vi "split and resample.vi"(9 "real zero index":i32=225, 10 "B field array":dbl[](array[numeric]), 11 "cond":T1(graph)) -> (0 "resampled number of curves":i32, 1 "new B field\noffset and multiplier":cluster{"N1":dbl, dbl}, 2 "resampled B":dbl[](array[numeric]), 3 "resampled cond":T1(graph))   [LabVIEW 2016, in "Tranconductance SM.lvclass"]
uses:
  Tranconductance SM.lvclass
  <userlib>/LevyLab/XY Utilities/Typedefs/Interpolation Configuration--cluster.ctl
  <userlib>/LevyLab/XY Utilities/subVIs/Interpolate (single).vi
  <userlib>/LevyLab/XY Utilities/xy_utilities.lvlib
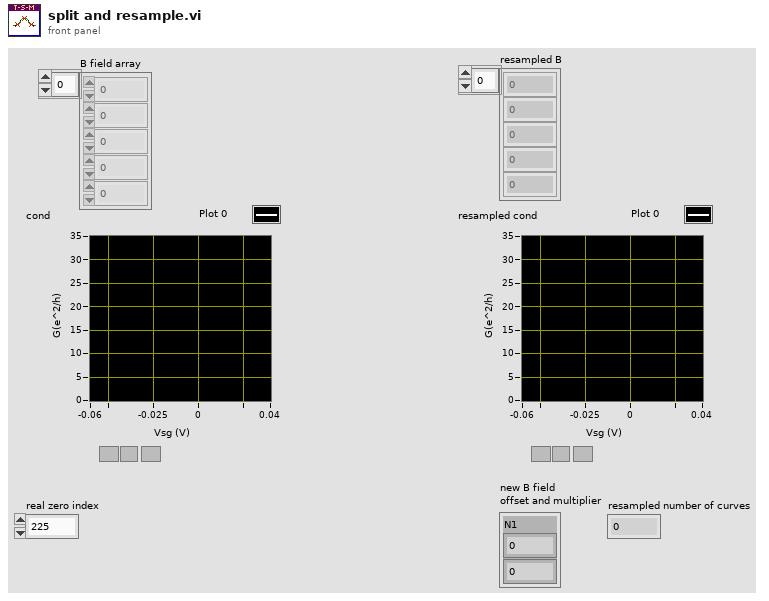
[diagram p1: front panel]
types:
  T1 = cluster{"Vfast":dbl[], "Decimated Array":dbl[]}[]
  T2 = typedef "xy_utilities.lvlib/Interpolation Configuration--cluster.ctl" = cluster{"X Low":dbl, "X High":dbl, "X Step":dbl, "Fake Point":dbl}
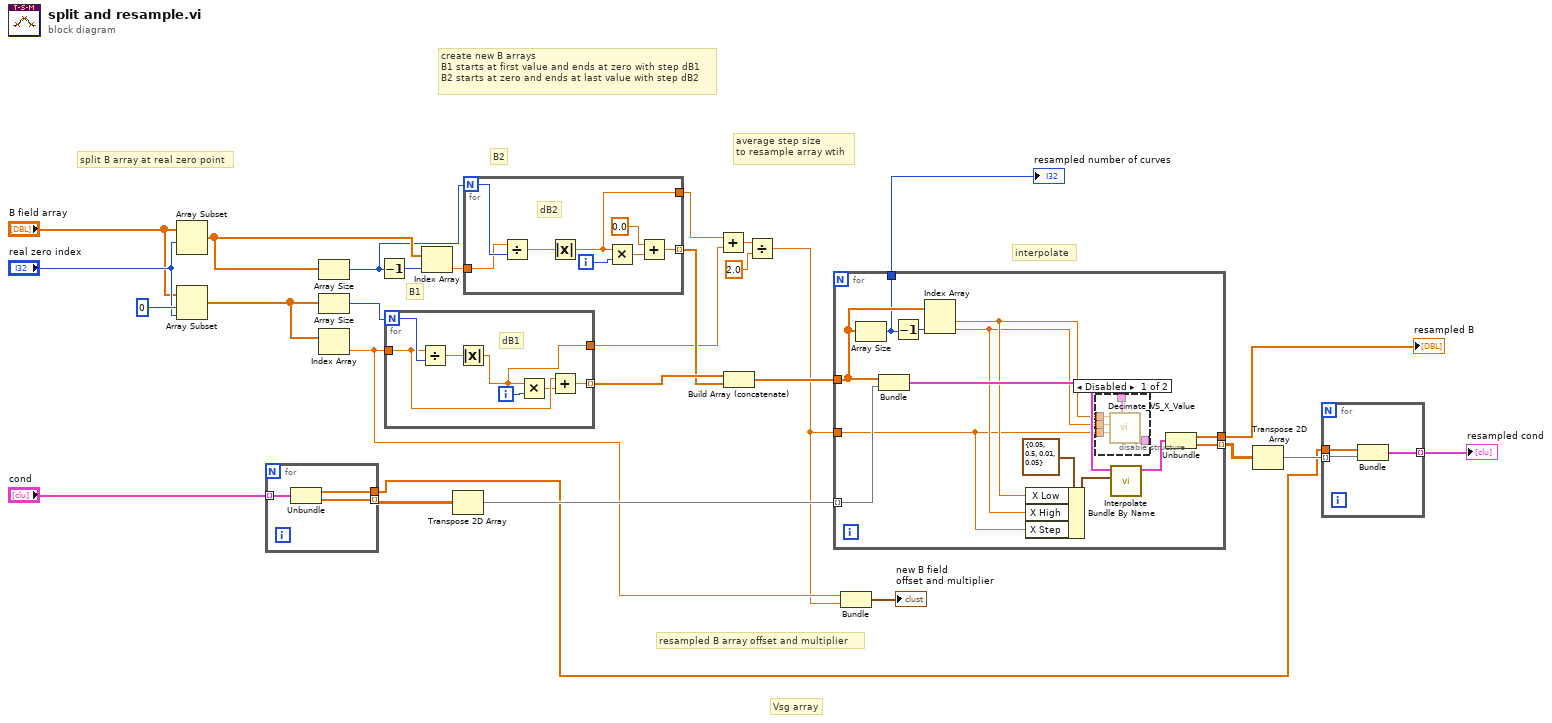
[diagram p0: block diagram]
diagram:
  # "average step size \nto resample array wtih"
  # "Vsg array"
  # "resampled B array offset and multiplier"
  # "interpolate"
  # "B1"
  # "B2"
  # "create new B arrays\nB1 starts at first value and ends at zero with step dB1\nB2 starts at zero and ends at last value with step dB2"
  # "split B array at real zero point"
  n1 = Array Subset(array="B field array", index="real zero index") -> (w23:dbl[])  [unwired: 1 in]
  n2 = Array Subset(array="B field array", index=0, length="real zero index") -> (w24:dbl[])
  n3 = for {
    tunnel: "cond" -> [w31] mode=indexing
    tunnel: [w30] -> w16 mode=indexing
    tunnel: [w29] -> w4
    n4 = Unbundle(w31) -> ("Vfast"=w29:dbl[], "Decimated Array"=w30:dbl[])
  }
  n5 = Array Size(array=w23) -> (size(s)=w21:i32)
  n6 = Array Size(array=w24) -> (size(s)=w25:i32)
  n7 = Index Array(array=w24) -> (element=w7:dbl)  [unwired: 1 in]
  n8 = Decrement(x=w21) -> (x-1=w20:i32)
  n9 = for {
    N: w25 -> [w38]
    tunnel: w7 -> [w36]
    tunnel: [w33] -> w19 mode=indexing
    tunnel: [w32] -> w12
    i -> [w35]
    # "dB1"
    n10 = Divide(x=w36, y=w38) -> (x/y=w37:dbl)
    n11 = Absolute Value(x=w37) -> (abs(x)=w32:dbl)
    n12 = Multiply(x=w32, y=w35) -> (x*y=w34:dbl)
    n13 = Add(x=w36, y=w34) -> (x+y=w33:dbl)
  }
  n14 = Index Array(array=w23, index=w20) -> (element=w22:dbl)
  n15 = Transpose 2D Array(2D array=w16) -> (transposed array=w15:dbl[][])
  n16 = for {
    N: w21 -> [w46]
    tunnel: w22 -> [w44]
    tunnel: [w41] -> w18 mode=indexing
    tunnel: [w39] -> w13
    i -> [w43]
    # "dB2"
    n17 = Divide(x=w44, y=w46) -> (x/y=w45:dbl)
    n18 = Absolute Value(x=w45) -> (abs(x)=w39:dbl)
    n19 = Multiply(x=w39, y=w43) -> (x*y=w42:dbl)
    n20 = Add(x=0.0, y=w42) -> (x+y=w41:dbl)
  }
  n21 = Add(x=w13, y=w12) -> (x+y=w11:dbl)
  n22 = Build Array (concatenate)(w19, w18) -> (w14:dbl[])
  n23 = Divide(x=w11, y=2.0) -> (x/y=w6:dbl)
  n24 = for {
    tunnel: w15 -> [w59] mode=indexing
    tunnel: w14 -> [w58]
    tunnel: w6 -> [w47]
    tunnel: [w56] -> w8
    tunnel: [w55] -> w9 mode=indexing
    tunnel: [w54] -> w1
    n25 = Array Size(array=w58) -> (size(s)=w54:i32)
    n26 = Bundle(w58, w59) -> (w53:cluster{dbl[], dbl[]})  [unwired: 1 in]
    n27 = Decrement(x=w54) -> (x-1=w57:i32)
    n28 = Index Array(array=w58, index #2=w57) -> (element #1=w49:dbl, element #2=w48:dbl)  [unwired: 1 in]
    n29 = Bundle By Name(cluster=T2 {"X Low"=0.05, "X High"=0.5, "X Step"=0.01, "Fake Point"=0.05} ("Configure"), "X Low"=w49, "X High"=w48, "X Step"=w47) -> (w50:T2)
    n30 = disable-structure shown="Disabled" {
      disable-tunnel: w53 -> [w64 _]
      disable-tunnel: [w63 _] -> _
      disable-tunnel: w49 -> [w62 _]
      disable-tunnel: w48 -> [w61 _]
      disable-tunnel: w47 -> [w60 _]
      frame Disabled {
        n31 = call <userlib>:"Decimate_VS_X_Value.vi"("XY Graph kind 1"=w64, "X Step"=w60, "X High"=w61, "X Low"=w62) -> ("Interpolated"=w63:cluster{dbl[], dbl[]})  [unwired: 6 in, 1 out]
      }
      frame Enabled {
      }
    }
    n32 = call-poly <userlib>:"Interpolate.vi"("Configure"=w50, "XY-data"=w53) -> ("Interpolated XY-data out"=w52:cluster{"X-array":dbl[], "Y-array":dbl[]})  [unwired: 8 in, 1 out]
    n33 = Unbundle(w52) -> ("X-array"=w56:dbl[], "Y-array"=w55:dbl[])
  }
  "resampled B" <- w8
  "resampled number of curves" <- w1
  n34 = Bundle("N1"=w7, w6) -> (→"new B field\noffset and multiplier":cluster{"N1":dbl, dbl})  [unwired: 1 in]
  n35 = Transpose 2D Array(2D array=w9) -> (transposed array=w5:dbl[][])
  n36 = for {
    tunnel: w5 -> [w66] mode=indexing
    tunnel: w4 -> [w67]
    tunnel: [w65] -> w3 mode=indexing
    n37 = Bundle("Vfast"=w67, w66) -> (w65:cluster{"Vfast":dbl[], dbl[]})  [unwired: 1 in]
  }
  "resampled cond" <- w3
